vi "DeleteCells.vi"(0 "SingleValCol in":refnum<class "SingleValCol.lvclass">, 5 "Cell Position":T1, 9 "Table CtlRef In":refnum<vi>, 11 "error in (no error)":errorcluster, 12 "# Rows":i32) -> (4 "SingleValCol out":refnum<class "SingleValCol.lvclass">, 10 "Table CtlRef Out":refnum<vi>, 15 "error out":errorcluster)   [LabVIEW 2013, in "SingleValCol.lvclass"]
doc: "Intended to be used as part of Delete Row(s) function, this method only shifts formatting. Values can be more efficiently deleted by row with array functions.\n\nThe funcitonality was made column-specific so that SingleVal can be handled appropriately."
uses:
  SingleValCol.lvclass
  <vilib>/Utility/miscctls.llb/LVRowAndColumnTypeDef.ctl
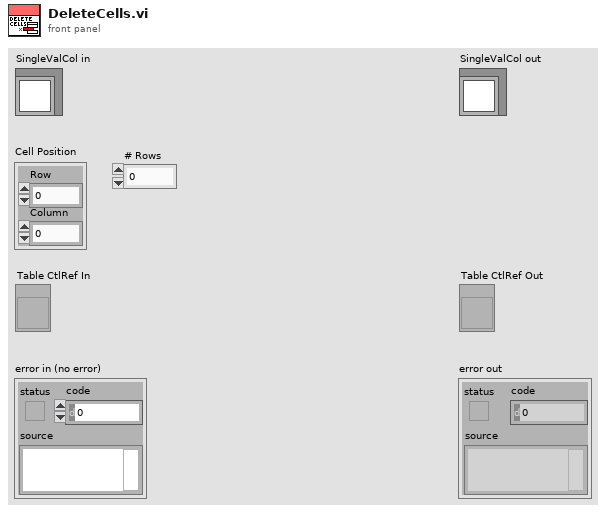
[diagram p1: front panel]
types:
  T1 = typedef "LVRowAndColumnTypeDef.ctl" = cluster{"Row":i32, "Column":i32}
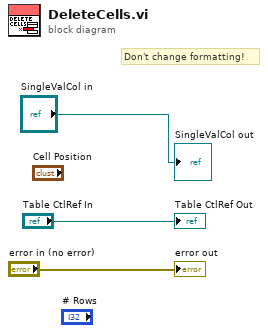
[diagram p0: block diagram]
diagram:
  # "Don't change formatting!"
  "error out" <- "error in (no error)"
  "SingleValCol out" <- "SingleValCol in"
  "Table CtlRef Out" <- "Table CtlRef In"
